vi "Inst_DS360.vi"(8 "error in":errorcluster, 10 "All Message Queues in":T1, 11 "Prueba10 in":refnum<class "Prueba10.lvclass">) -> (0 "error out":errorcluster)   [LabVIEW 2019, in "Prueba10.lvclass"]
uses:
  Prueba10.lvclass
  QMH/Message Queue/All Message Queues.ctl
  QMH/Message Queue/Message Cluster.ctl
  Prueba10.lvclass/Prueba10.ctl
  ClusterGEN.ctl
  <vilib>/Utility/error.llb/Error Cluster From Error Code.vi
  QMH/Message Queue/Enqueue Message (Single).vi
  <vilib>/ErrorRing/Error Ring.xnode
  QMH/Message Queue/Message Queue.lvlib
  Instrumento/DS360/DS360.lvclass
panel:
  out "All States":string[](array[string])
  out "Actual State":string
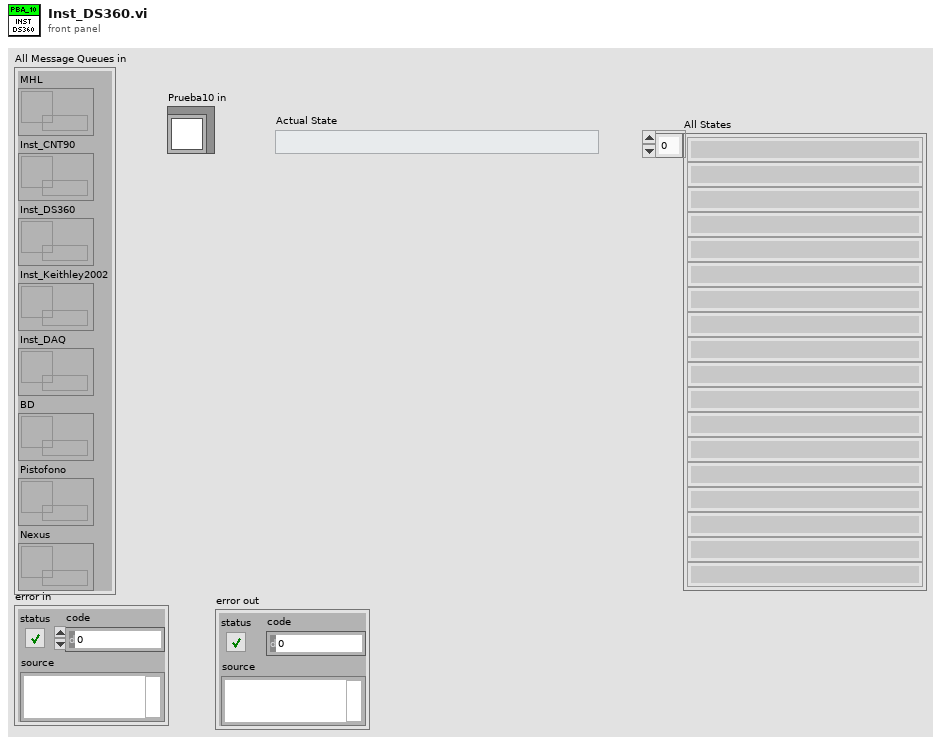
[diagram p1: front panel]
types:
  T1 = typedef "Message Queue.lvlib/All Message Queues.ctl" = cluster{"MHL":refnum<queue>, "Inst_CNT90":refnum<queue>, "Inst_DS360":refnum<queue>, "Inst_Keithley2002":refnum<queue>, "Inst_DAQ":refnum<queue>, "BD":refnum<queue>, "Pistofono":refnum<queue>, "Nexus":refnum<queue>}
  T2 = typedef "Prueba10.lvclass/ClusterGEN.ctl" = cluster{"frec":dbl, "amp":dbl}
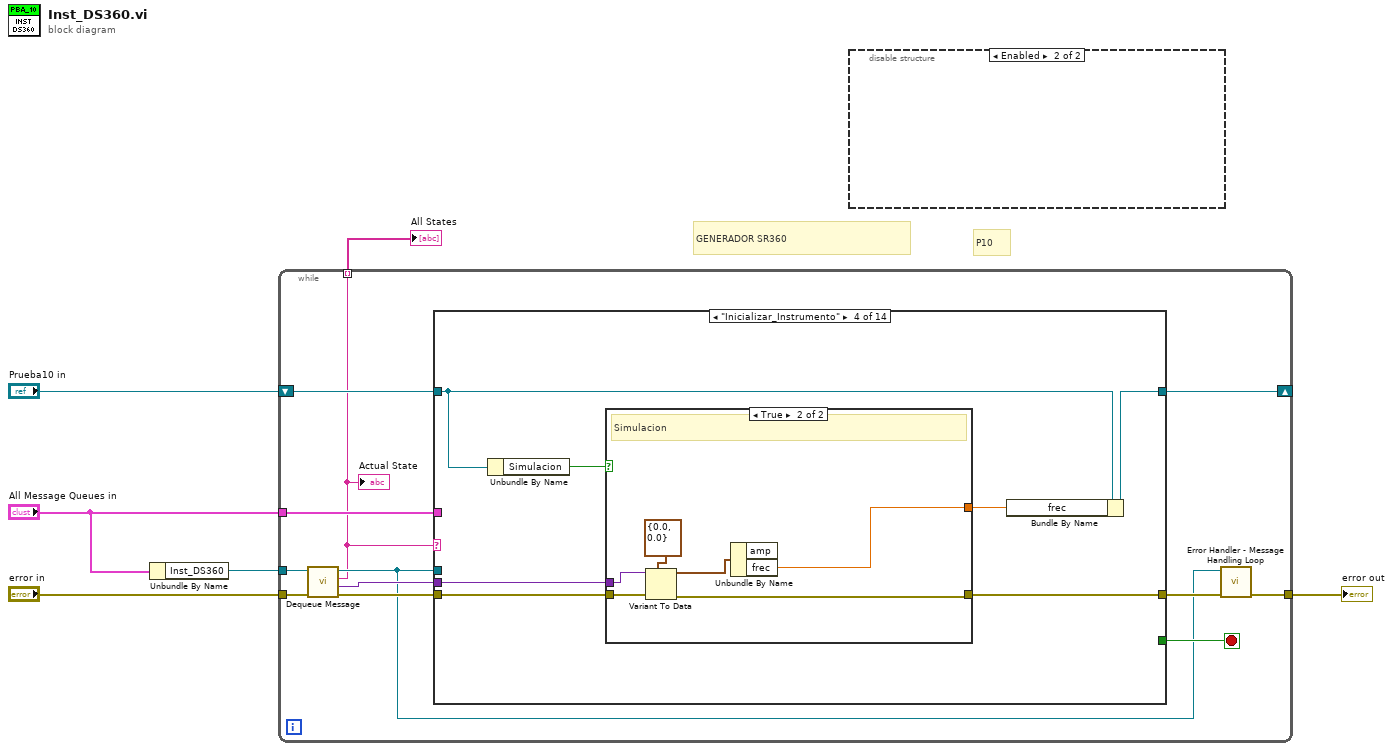
[diagram p0: block diagram]
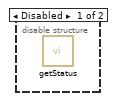
[diagram p2: hidden frame]
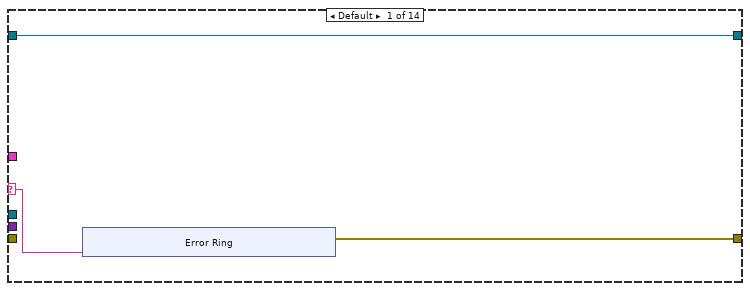
[diagram p3: hidden frame]
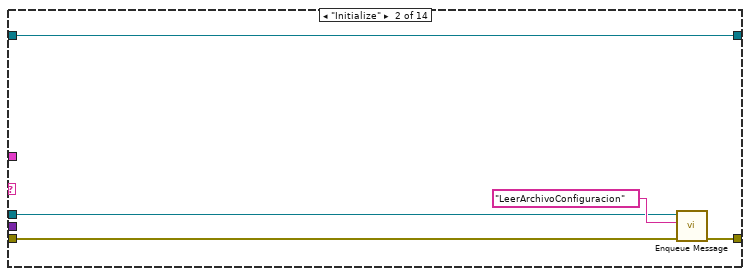
[diagram p4: hidden frame]
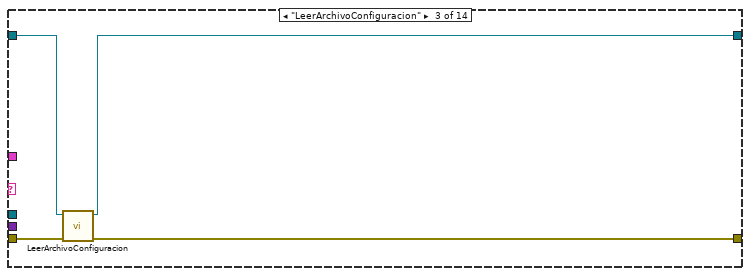
[diagram p5: hidden frame]
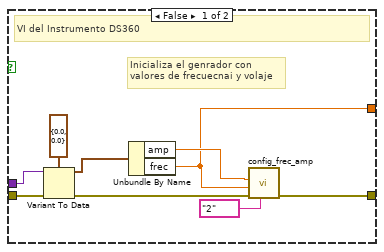
[diagram p6: hidden frame]
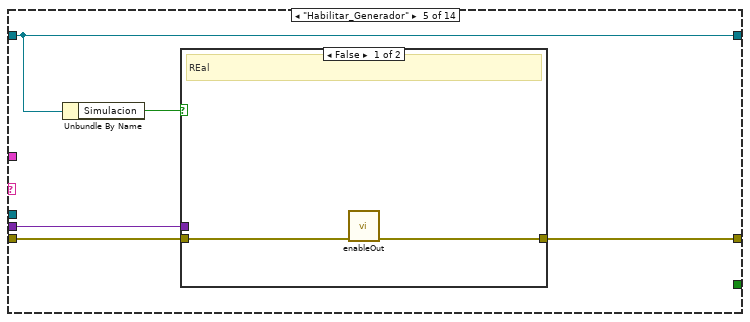
[diagram p7: hidden frame]
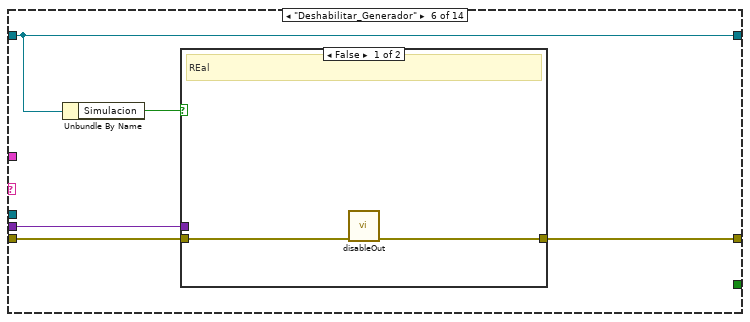
[diagram p9: hidden frame]
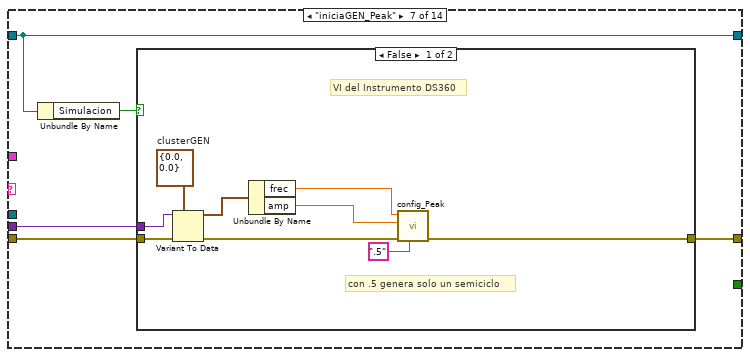
[diagram p11: hidden frame]
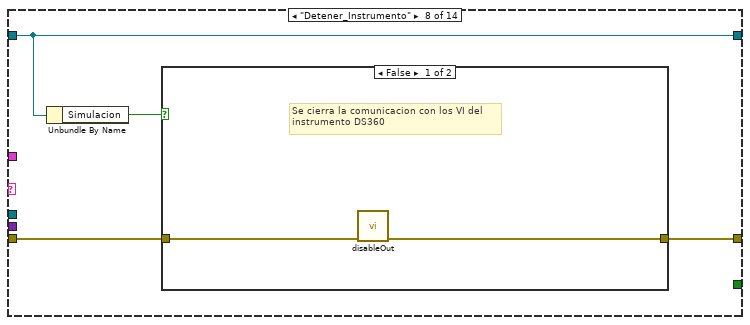
[diagram p13: hidden frame]
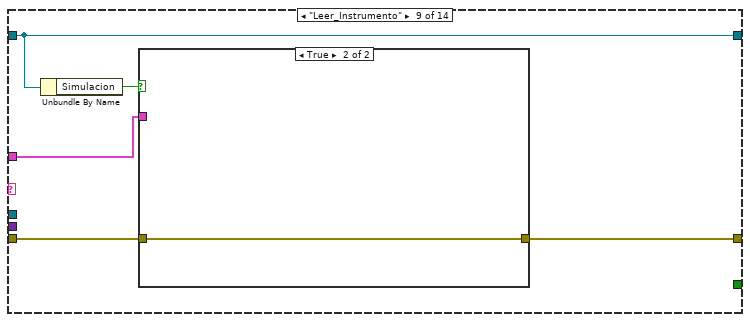
[diagram p15: hidden frame]
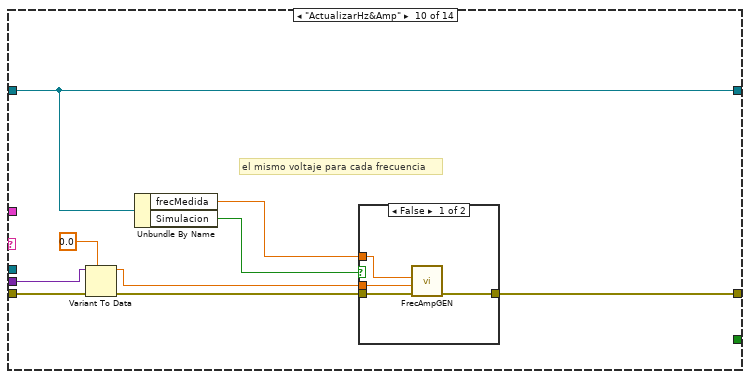
[diagram p17: hidden frame]
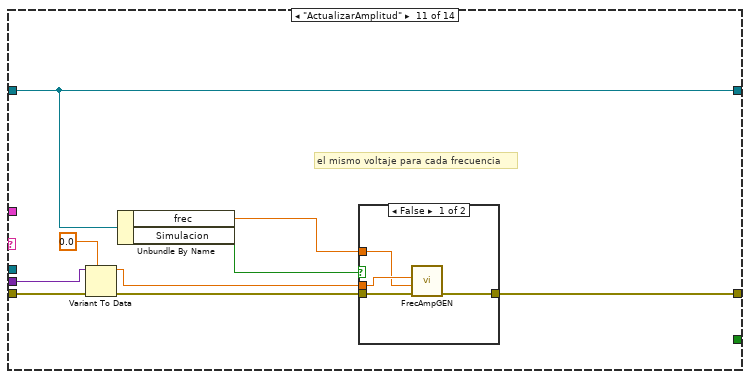
[diagram p19: hidden frame]
diagram:
  # "P10"
  # "GENERADOR SR360"
  n1 = Unbundle By Name("All Message Queues in") -> ("Inst_DS360"=w4:refnum<queue>)
  n2 = while {
    tunnel: "error in" -> [w18]
    tunnel: w4 -> [w17]
    tunnel: "All Message Queues in" -> [w16]
    tunnel: [w9] -> w2
    shift-right: [w12] -> _
    shift-left: "Prueba10 in" -> [w15]
    tunnel: [w7] -> w1 mode=indexing
    stop <- w11 stop-if-true
    n3 = call "Dequeue Message.vi"("error in (no error)"=w18, "Message Queue"=w17) -> ("error out"=w13:errorcluster, "Message Data"=w14:variant, "Message"=w7:string, "dup Message Queue"=w8:refnum<queue>)  [unwired: 6 in]
    "Actual State" <- w7
    n4 = case shown="\"Inicializar_Instrumento\"" w7 {
      selector: w7 -> [w21 _ _ _ _ _ _ _ _ _ _ _ w147 _]
      tunnel: w16 -> [_ _ _ _ _ _ _ _ w101 _ _ _ w146 _]
      tunnel: w15 -> [w19 w33 w34 w42 w63 w71 w78 w93 w100 w109 w123 w136 w154 w156]
      tunnel: w8 -> [_ w29 _ _ _ _ _ _ _ _ _ _ _ w158]
      tunnel: w14 -> [_ _ _ w41 w62 w70 w77 _ _ w110 w124 w137 w151 _]
      tunnel: w13 -> [_ w30 w36 w40 w61 w69 w76 w91 w102 w111 w125 w138 w152 w159]
      tunnel: [w20 w31 w37 w44 w60 w68 w80 w94 w98 w113 w127 w140 w149 w155] -> w10
      tunnel: [w19 w33 w35 w39 w63 w71 w78 w93 w100 w109 w123 w136 w154 w156] -> w12
      tunnel: [_ _ _ _ _ _ _ _ _ _ _ _ _ TRUE] -> w11
      frame Default {
        n5 = xnode "Error Ring"("parameter 0"=w21) -> ("error out"=w20:errorcluster)
      }
      frame "Initialize" {
        n6 = call-poly "Enqueue Message.vi"("error in (no error)"=w30, "Message"="LeerArchivoConfiguracion", "Message Queue"=w29) -> ("error out"=w31:errorcluster)  [unwired: 7 in, 1 out]
      }
      frame "LeerArchivoConfiguracion" {
        n7 = call "LeerArchivoConfiguracion.vi"("error in"=w36, "Prueba10 in"=w34) -> ("error out"=w37:errorcluster, "Prueba10 out"=w35:refnum<class "Prueba10.lvclass">)  [unwired: 8 in]
      }
      frame "Inicializar_Instrumento" {
        n8 = Unbundle By Name(w42) -> ("Simulacion"=w43:bool)
        n9 = case shown="True" w43 {
          tunnel: [w52 w57] -> w44
          tunnel: w40 -> [w53 w59]
          tunnel: w41 -> [w50 w58]
          tunnel: [w47 w54] -> w38
          frame False {
            # "Inicializa el genrador con \nvalores de frecuecnai y volaje"
            # "VI del Instrumento DS360"
            n10 = Variant To Data(error in=w53, type=T2 {"frec"=0.0, "amp"=0.0} ("clusterGEN"), Variant=w50) -> (data=w49:T2, error out=w51:errorcluster)
            n11 = Unbundle By Name(w49) -> ("amp"=w48:dbl, "frec"=w47:dbl)
            n12 = call "config_frec_amp.vi"("Impedancia"="2", "error in (no error)"=w51, "Frec (Hz)"=w47, "Amplitud (Vrms)"=w48) -> ("error out"=w52:errorcluster)  [unwired: 6 in, 1 out]
          }
          frame True {
            # "Simulacion"
            n13 = Variant To Data(error in=w59, type=T2 {"frec"=0.0, "amp"=0.0} ("clusterGEN"), Variant=w58) -> (data=w55:T2, error out=w57:errorcluster)
            n14 = Unbundle By Name(w55) -> ("frec"=w54:dbl)  [unwired: 1 out]
          }
        }
        n15 = Bundle By Name(cluster=w42, "frec"=w38) -> (w39:refnum<class "Prueba10.lvclass">)
      }
      frame "Habilitar_Generador" {
        n16 = Unbundle By Name(w63) -> ("Simulacion"=w64:bool)
        n17 = case shown="False" w64 {
          tunnel: w61 -> [w66 w67]
          tunnel: w62 -> [_ _]
          tunnel: [w65 w67] -> w60
          frame False {
            # "REal"
            n18 = call "enableOut.vi"("error in (no error)"=w66) -> ("error out"=w65:errorcluster)  [unwired: 9 in, 1 out]
          }
          frame True {
            # "Simulacion"
          }
        }
      }
      frame "Deshabilitar_Generador" {
        n19 = Unbundle By Name(w71) -> ("Simulacion"=w72:bool)
        n20 = case shown="False" w72 {
          tunnel: w69 -> [w74 w75]
          tunnel: w70 -> [_ _]
          tunnel: [w73 w75] -> w68
          frame False {
            # "REal"
            n21 = call "disableOut.vi"("error in (no error)"=w74) -> ("error out"=w73:errorcluster)  [unwired: 9 in, 1 out]
          }
          frame True {
            # "Simulacion"
          }
        }
      }
      frame "iniciaGEN_Peak" {
        n22 = Unbundle By Name(w78) -> ("Simulacion"=w79:bool)
        n23 = case shown="False" w79 {
          tunnel: [w84 w90] -> w80
          tunnel: w76 -> [w89 w90]
          tunnel: w77 -> [w88 _]
          frame False {
            w86 = T2 {"frec"=0.0, "amp"=0.0}  # clusterGEN
            # "con .5 genera solo un semiciclo"
            # "VI del Instrumento DS360"
            n24 = Variant To Data(error in=w89, type=w86, Variant=w88) -> (data=w87:T2, error out=w85:errorcluster)
            n25 = Unbundle By Name(w87) -> ("frec"=w83:dbl, "amp"=w82:dbl)
            n26 = call "config_Peak.vi"("tipo_ciclo"=".5", "error in (no error)"=w85, "Amplitud (Vrms)"=w82, "Frec (Hz)"=w83) -> ("error out"=w84:errorcluster)  [unwired: 6 in, 1 out]
          }
          frame True {
            # "Simulacion"
          }
        }
      }
      frame "Detener_Instrumento" {
        n27 = Unbundle By Name(w93) -> ("Simulacion"=w92:bool)
        n28 = case shown="False" w92 {
          tunnel: [w96 w97] -> w94
          tunnel: w91 -> [w95 w97]
          frame False {
            # "Se cierra la comunicacion con los VI del\ninstrumento DS360"
            n29 = call "disableOut.vi"("error in (no error)"=w95) -> ("error out"=w96:errorcluster)  [unwired: 9 in, 1 out]
          }
          frame True {
            # "Simulacion"
          }
        }
      }
      frame "Leer_Instrumento" {
        n30 = Unbundle By Name(w100) -> ("Simulacion"=w99:bool)
        n31 = case shown="True" w99 {
          tunnel: [w103 w104] -> w98
          tunnel: w102 -> [w103 w104]
          tunnel: w101 -> [_ _]
          frame False {
          }
          frame True {
          }
        }
      }
      frame "ActualizarHz&Amp" {
        # "el mismo voltaje para cada frecuencia"
        n32 = Variant To Data(error in=w111, type=0.0, Variant=w110) -> (data=w106:dbl, error out=w112:errorcluster)
        n33 = Unbundle By Name(w109) -> ("frecMedida"=w108:dbl, "Simulacion"=w105:bool)
        n34 = case shown="False" w105 {
          tunnel: [w117 w118] -> w113
          tunnel: w112 -> [w116 w118]
          tunnel: w108 -> [w115 _]
          tunnel: w106 -> [w114 _]
          frame False {
            n35 = call "FrecAmpGEN.vi"("error in (no error)"=w116, "Frec (Hz)"=w114, "Amplitud (Vrms)"=w115) -> ("error out"=w117:errorcluster)  [unwired: 7 in, 1 out]
          }
          frame True {
            # "Simlacion"
          }
        }
      }
      frame "ActualizarAmplitud" {
        # "el mismo voltaje para cada frecuencia"
        n36 = Variant To Data(error in=w125, type=0.0, Variant=w124) -> (data=w121:dbl, error out=w126:errorcluster)
        n37 = Unbundle By Name(w123) -> ("frec"=w119:dbl, "Simulacion"=w120:bool)
        n38 = case shown="False" w120 {
          tunnel: [w131 w132] -> w127
          tunnel: w126 -> [w130 w132]
          tunnel: w121 -> [w129 _]
          tunnel: w119 -> [w128 _]
          frame False {
            n39 = call "FrecAmpGEN.vi"("error in (no error)"=w130, "Frec (Hz)"=w128, "Amplitud (Vrms)"=w129) -> ("error out"=w131:errorcluster)  [unwired: 7 in, 1 out]
          }
          frame True {
            # "Simlacion"
          }
        }
      }
      frame "ActualizarFrecuencia" {
        # "el mismo voltaje para cada frecuencia"
        n40 = Variant To Data(error in=w138, type=0.0, Variant=w137) -> (data=w134:dbl, error out=w139:errorcluster)
        n41 = Unbundle By Name(w136) -> ("Simulacion"=w133:bool)
        n42 = case shown="False" w133 {
          tunnel: [w143 w144] -> w140
          tunnel: w139 -> [w142 w144]
          tunnel: w134 -> [w141 _]
          frame False {
            n43 = call "FrecAmpGEN.vi"("error in (no error)"=w142, "Frec (Hz)"=w141) -> ("error out"=w143:errorcluster)  [unwired: 8 in, 1 out]
          }
          frame True {
            # "Simlacion"
          }
        }
      }
      frame "Error" {
        n44 = Unbundle By Name(w146) -> ("MHL"=w145:refnum<queue>)
        n45 = Variant To Data(error in=w152, type=errorcluster {"status"=FALSE, "code"=0, "source"=""} ("error constant"), Variant=w151) -> (data=w148:errorcluster, error out=w150:errorcluster)
        n46 = call-poly "Enqueue Message.vi"("error in (no error)"=w150, "Message Data"=w148, "Message"=w147, "Message Queue"=w145) -> ("error out"=w149:errorcluster)  [unwired: 6 in, 1 out]
      }
      frame "Exit" {
        n47 = Release Queue(queue=w158, error in (no error)=w159) -> (error out=w155:errorcluster)  [unwired: 1 in, 2 out]
      }
    }
    n48 = call "Error Handler - Message Handling Loop.vi"("error in (no error)"=w10, "Message Queue"=w8) -> ("dup error in"=w9:errorcluster)  [unwired: 8 in, 1 out]
  }
  "error out" <- w2
  "All States" <- w1
  n49 = disable-structure shown="Enabled" {
    frame Disabled {
      n50 = call "getStatus.vi"() -> ()  [unwired: 9 in, 3 out]
    }
    frame Enabled {
    }
  }
